vi "Get reference to all controls.vi"(4 "error in (no error)":errorcluster) -> (0 "error out":errorcluster, 2 "Control references":T1(array[cluster]))   [LabVIEW 2019]
doc: "This VI gets a Reference to All Controls on the Front Panel of the VI which calls it. It returns a 2D array of All the References and Labels for Each Control."
panel:
  in  "GetClassIDTab":enum32{"Page 1", "Page 2"}(tab)
  in  "Cntrl Ref":refnum<vi>[](array[refnum])
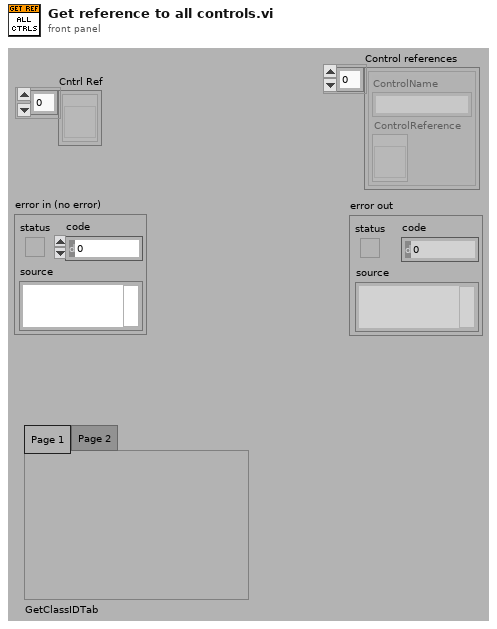
[diagram p1: front panel]
types:
  T1 = cluster{"ControlName":string, "ControlReference":refnum<vi>}[]
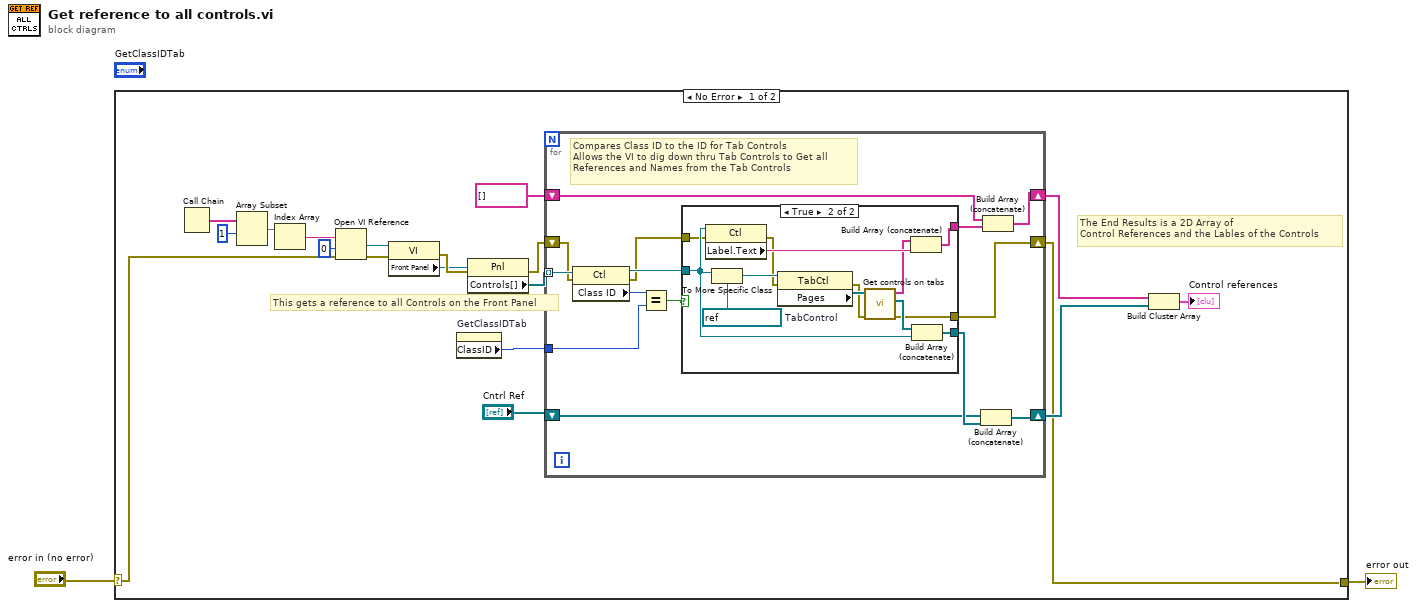
[diagram p0: block diagram]
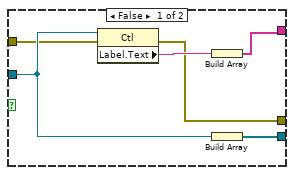
[diagram p2: hidden frame]
diagram:
  n1 = case shown="No Error" "error in (no error)" {
    selector: "error in (no error)" -> [w9 w55]
    tunnel: [w4 w55] -> w2
    frame No Error {
      # "The End Results is a 2D Array of \nControl References and the Lables of the Controls"
      # "This gets a reference to all Controls on the Front Panel"
      n2 = Call Chain() -> (call chain=w19:string[])
      n3 = Array Subset(array=w19, index=1) -> (w5:string[])  [unwired: 1 in]
      n4 = Index Array(array=w5) -> (element=w21:string)  [unwired: 1 in]
      n5 = Open VI Reference(vi path=w21, options=0, error in (no error)=w9) -> (vi reference=w14:refnum<vi>, error out=w8:errorcluster)  [unwired: 3 in]
      n6 = property class="VI"(reference=w14, error in=w8) -> (error out=w15:errorcluster, "Front Panel"=w12:refnum<vi>)  [unwired: 1 out]
      n7 = property on="GetClassIDTab" class="TabCtl (strict)"() -> ("ClassID"=w3:u32)  [unwired: 2 in, 2 out]
      n8 = property class="Pnl"(reference=w12, error in=w15) -> (error out=w7:errorcluster, "Controls[]"=w13:refnum<vi>[])  [unwired: 1 out]
      n9 = for {
        tunnel: w13 -> [w35] mode=indexing
        shift-right: [w27] -> w16
        shift-left: string[] [] -> [w29]
        shift-right: [w32] -> w17
        shift-left: "Cntrl Ref" -> [w30]
        shift-right: [w23] -> w4
        shift-left: w7 -> [w25]
        tunnel: w3 -> [w22]
        # "Compares Class ID to the ID for Tab Controls\nAllows the VI to dig down thru Tab Controls to Get all \nReferences and Names from the Tab Controls"
        n10 = property class="Ctl"(reference=w35, error in=w25) -> (reference out=w26:refnum<vi>, error out=w24:errorcluster, "Class ID"=w34:u32)
        n11 = Equal?(x=w34, y=w22) -> (x = y?=w33:bool)
        n12 = case shown="True" w33 {
          tunnel: w26 -> [w40 w51]
          tunnel: [w41 w53] -> w31
          tunnel: [w38 w49] -> w28
          tunnel: w24 -> [w37 w48]
          tunnel: [w36 w42] -> w23
          frame False {
            n13 = property class="Ctl"(reference=w40, error in=w37) -> (error out=w36:errorcluster, "Label.Text"=w39:string)  [unwired: 1 out]
            n14 = Build Array(w39) -> (w38:string[])
            n15 = Build Array(w40) -> (w41:refnum<vi>[])
          }
          frame True {
            w54 = refnum<vi> refnum  # TabControl
            n16 = property class="Ctl"(reference=w51, error in=w48) -> (error out=w44:errorcluster, "Label.Text"=w50:string)  [unwired: 1 out]
            n17 = To More Specific Class(target class=w54, reference=w51) -> (specific class reference=w52:refnum<vi>)  [unwired: 1 in, 1 out]
            n18 = property class="TabCtl"(reference=w52, error in=w44) -> (error out=w43:errorcluster, "Pages"=w45:refnum<vi>[])  [unwired: 1 out]
            n19 = call "Get controls on tabs.vi"("error in"=w43, "Pages"=w45) -> ("error out"=w42:errorcluster, "Cntrl Ref"=w46:refnum<vi>[], "Cntrl Labels"=w47:string[])  [unwired: 7 in]
            n20 = Build Array (concatenate)(w47, w50) -> (w49:string[])
            n21 = Build Array (concatenate)(w46, w51) -> (w53:refnum<vi>[])
          }
        }
        n22 = Build Array (concatenate)(w30, w31) -> (w32:refnum<vi>[])
        n23 = Build Array (concatenate)(w29, w28) -> (w27:string[])
      }
      n24 = Build Cluster Array(w16, w17) -> (→"Control references":cluster{string, refnum<vi>}[])
    }
    frame Error {
    }
  }
  "error out" <- w2
